vi "how long is resp data.vi"(7 "resp (t) req(f)":bool, 10 "first (1/4) bytes":u8[](array[numeric]), 11 "func":u8) -> (3 "bytes in PDU  after func":i32)   [LabVIEW 2021, in "RTU Data Unit.lvclass"]
uses:
  RTU Data Unit.lvclass
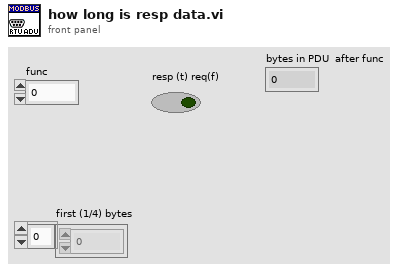
[diagram p1: front panel]
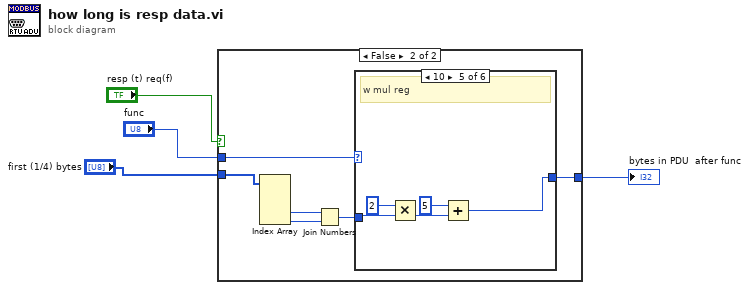
[diagram p0: block diagram]
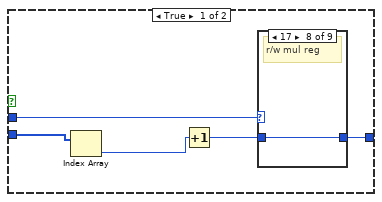
[diagram p2: hidden frame]
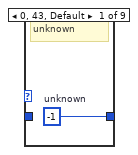
[diagram p3: hidden frame]
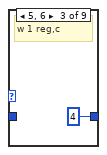
[diagram p5: hidden frame]
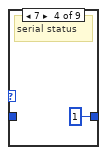
[diagram p6: hidden frame]
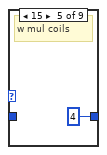
[diagram p7: hidden frame]
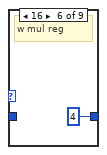
[diagram p8: hidden frame]
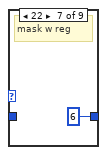
[diagram p9: hidden frame]
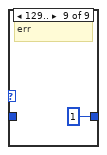
[diagram p10: hidden frame]
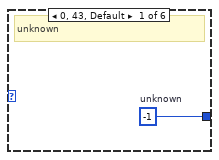
[diagram p11: hidden frame]
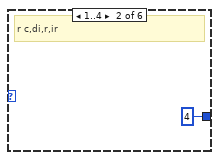
[diagram p12: hidden frame]
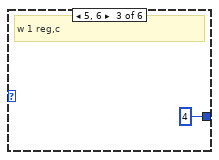
[diagram p13: hidden frame]
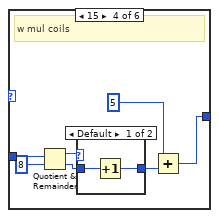
[diagram p14: hidden frame]
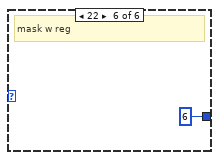
[diagram p16: hidden frame]
diagram:
  n1 = case shown="False" "resp (t) req(f)" {
    tunnel: [w9 w24] -> w4
    tunnel: "func" -> [w8 w23]
    tunnel: "first (1/4) bytes" -> [w6 w22]
    frame True {
      n2 = Index Array(array=w6) -> (element=w5:u8)  [unwired: 1 in]
      n3 = Increment(x=w5) -> (x+1=w7:u8)
      n4 = case shown="17" w8 {
        tunnel: [w10 w11 4 ("bytes to read") 1 ("bytes to read") 4 ("bytes to read") 4 ("bytes to read") 6 ("bytes to read") w17 1 ("bytes to read")] -> w9
        tunnel: w7 -> [_ w11 _ _ _ _ _ w17 _]
        frame 0, 43, Default {
          w10 = -1  # unknown
          # "unknown"
        }
        frame 1..4 {
          # "r c,di,r,ir"
        }
        frame 5, 6 {
          # "w 1 reg,c"
        }
        frame 7 {
          # "serial status"
        }
        frame 15 {
          # "w mul coils"
        }
        frame 16 {
          # "w mul reg"
        }
        frame 22 {
          # "mask w reg"
        }
        frame 23 {
          # "r/w mul reg"
        }
        frame 129.. {
          # "err"
        }
      }
    }
    frame False {
      n5 = Index Array(array=w22) -> (element #3=w21:u8, element #4=w20:u8)  [unwired: 4 in, 2 out]
      n6 = Join Numbers(hi=w21, lo=w20) -> ((hi.lo)=w19:u16)
      n7 = case shown="10" w23 {
        tunnel: [w25 4 ("bytes to read") 4 ("bytes to read") w29 w40 6 ("bytes to read")] -> w24
        tunnel: w19 -> [_ _ _ w34 w42 _]
        frame 0, 43, Default {
          w25 = -1  # unknown
          # "unknown"
        }
        frame 1..4 {
          # "r c,di,r,ir"
        }
        frame 5, 6 {
          # "w 1 reg,c"
        }
        frame 15 {
          # "w mul coils"
          n8 = Quotient & Remainder(x=w34, y=u16 8) -> (x-y*floor(x/y)=w32:u16, floor(x/y)=w30:u16)
          n9 = case shown="Default" w32 {
            tunnel: [w35 w37] -> w31
            tunnel: w30 -> [w36 w37]
            frame Default {
              n10 = Increment(x=w36) -> (x+1=w35:u16)
            }
            frame 0 {
            }
          }
          n11 = Add(x=u16 5, y=w31) -> (x+y=w29:u16)
        }
        frame 16 {
          # "w mul reg"
          n12 = Multiply(x=u16 2, y=w42) -> (x*y=w39:u16)
          n13 = Add(x=u16 5, y=w39) -> (x+y=w40:u16)
        }
        frame 22 {
          # "mask w reg"
        }
      }
    }
  }
  "bytes in PDU  after func" <- w4
